vi "Get Enabled State.vi"(1 "Enabled?":bool) -> (0 "State":T1(ring))   [LabVIEW 2020, in "Output Sequencer.lvlib" / "Settings UI.lvclass"]
uses:
  Settings UI.lvclass
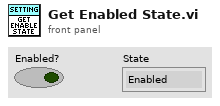
[diagram p1: front panel]
types:
  T1 = enum8{"Enabled", "Disabled", "Disabled and Grayed Out"}
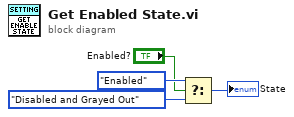
[diagram p0: block diagram]
diagram:
  n1 = Select(t=T1."Enabled" ("Disabled"), s="Enabled?", f=T1."Disabled and Grayed Out" ("Disabled")) -> (s? t:f=→"State":T1)
